vi "Setup-Input-Output-DAQmx.vi"(9 "Sample Rate":dbl=41200.0, 10 "samples per channel":i32=1000, 11 "Accel. 2":bool) -> (0 "error out":errorcluster, 2 "Output task":refnum<k21>, 3 "Input Task":refnum<k21>)   [LabVIEW 2022 SP3]
uses:
  <vilib>/Utility/error.llb/DialogType.ctl
  <vilib>/DAQmx/create/channels.llb/DAQmx Create Channel (AI-Acceleration-Accelerometer).vi
  <vilib>/DAQmx/create/channels.llb/DAQmx Create Channel (AO-Voltage-Basic).vi
  <vilib>/DAQmx/configure/timing.llb/DAQmx Timing (Sample Clock).vi
  <vilib>/DAQmx/configure/trigger.llb/DAQmx Start Trigger (Digital Edge).vi
panel:
  in  "source":tag
  in  "edge":i32(ring)=10280 items=["Rising"=10280, "Falling"=10171]
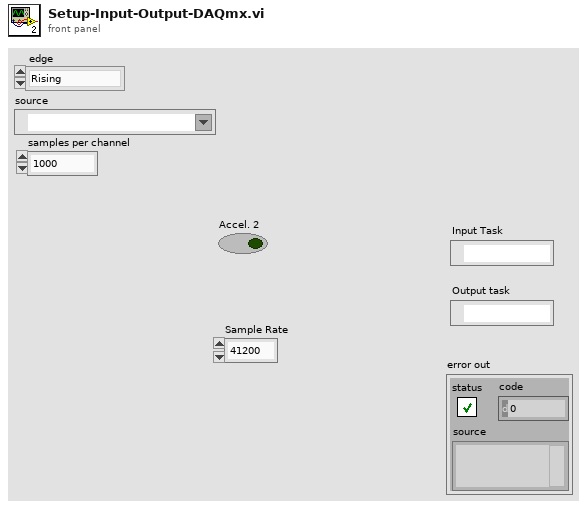
[diagram p1: front panel]
types:
  T1 = typedef "DialogType.ctl" = u16
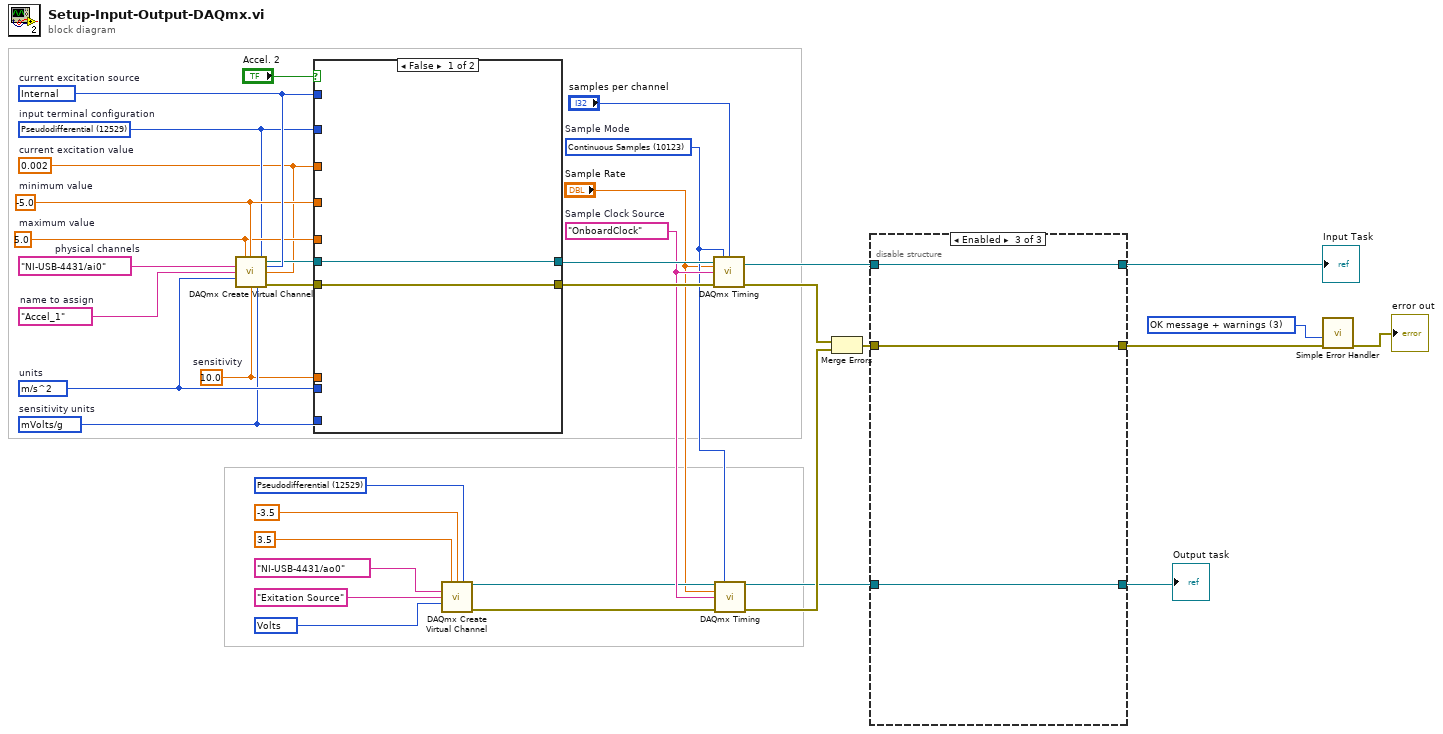
[diagram p0: block diagram]
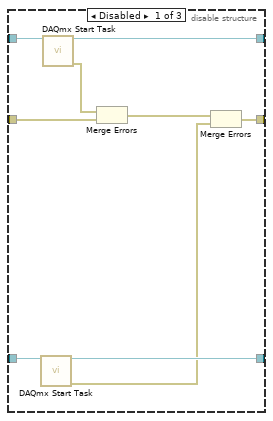
[diagram p2: hidden frame]
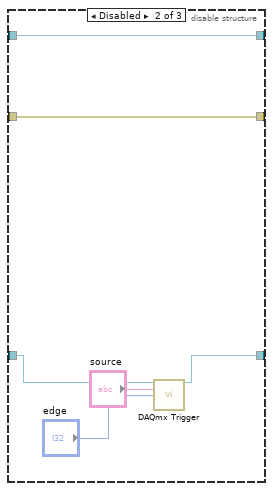
[diagram p3: hidden frame]
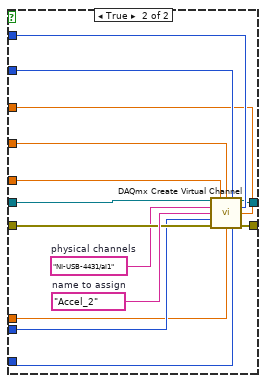
[diagram p4: hidden frame]
diagram:
  w6 = T1 3 items=["no dialog", "OK message", "continue or stop message", "OK message + warnings", "continue/stop + warnings"] ("type of dialog (OK msg:1)")
  w24 = 12529 items=["Default"=-1, "RSE"=10083, "Differential"=10106, "Pseudodifferential"=12529] ("output terminal configuration")
  w22 = 10348 items=["Volts"=10348, "From Custom Scale"=10065] ("units")
  w28 = 12509 items=["mVolts/g"=12509, "Volts/g"=12510]  # sensitivity units
  w20 = 10.0  # sensitivity
  w27 = 0.002  # current excitation value
  w35 = 10200 items=["Internal"=10200, "External"=10167, "None"=10230]  # current excitation source
  w29 = tag "NI-USB-4431/ai0"  # physical channels
  w17 = tag "OnboardClock"  # Sample Clock Source
  w16 = 10123 items=["Finite Samples"=10178, "Continuous Samples"=10123, "Hardware Timed Single Point"=12522]  # Sample Mode
  w31 = 12529 items=["default"=-1, "RSE"=10083, "NRSE"=10078, "Differential"=10106, "Pseudodifferential"=12529]  # input terminal configuration
  w34 = -5.0  # minimum value
  w33 = 5.0  # maximum value
  w37 = "Accel_1"  # name to assign
  w32 = 12470 items=["g"=10186, "m/s^2"=12470, "in/s^2"=12471, "From Custom Scale"=10065]  # units
  n1 = call-poly <vilib>:"DAQmx Create Virtual Channel.vi"("maximum value"=w33, "minimum value"=w34, "input terminal configuration"=w31, "physical channels"=w29, "current excitation source"=w35, "name to assign"=w37, "current excitation value"=w27, "units"=w32, "sensitivity"=w20, "sensitivity units"=w28) -> ("task out"=w30:refnum<k21>, "error out"=w36:errorcluster)  [unwired: 4 in]
  n2 = case shown="False" "Accel. 2" {
    tunnel: w36 -> [w39 w52]
    tunnel: w35 -> [_ w51]
    tunnel: w34 -> [_ w50]
    tunnel: w33 -> [_ w49]
    tunnel: w32 -> [_ w48]
    tunnel: w31 -> [_ w47]
    tunnel: w30 -> [w38 w46]
    tunnel: w28 -> [_ w44]
    tunnel: w27 -> [_ w43]
    tunnel: w20 -> [_ w42]
    tunnel: [w39 w41] -> w19
    tunnel: [w38 w40] -> w18
    frame False {
    }
    frame True {
      w45 = tag "NI-USB-4431/ai1"  # physical channels
      w53 = "Accel_2"  # name to assign
      n3 = call-poly <vilib>:"DAQmx Create Virtual Channel.vi"("task in"=w46, "maximum value"=w49, "minimum value"=w50, "input terminal configuration"=w47, "physical channels"=w45, "current excitation source"=w51, "name to assign"=w53, "current excitation value"=w43, "units"=w48, "error in"=w52, "sensitivity"=w42, "sensitivity units"=w44) -> ("task out"=w40:refnum<k21>, "error out"=w41:errorcluster)  [unwired: 2 in]
    }
  }
  n4 = call-poly <vilib>:"DAQmx Create Virtual Channel.vi"("maximum value"=3.5, "minimum value"=-3.5, "output terminal configuration"=w24, "physical channels"=tag "NI-USB-4431/ao0", "name to assign"="Exitation Source", "units"=w22) -> ("task out"=w14:refnum<k21>, "error out"=w15:errorcluster)  [unwired: 8 in]
  n5 = call-poly <vilib>:"DAQmx Timing.vi"("task/channels in"=w18, "sample mode"=w16, "samples per channel"="samples per channel", "rate"="Sample Rate", "source"=w17, "error in"=w19) -> ("task out"=w10:refnum<k21>, "error out"=w5:errorcluster)  [unwired: 8 in]
  n6 = call-poly <vilib>:"DAQmx Timing.vi"("task/channels in"=w14, "sample mode"=w16, "rate"="Sample Rate", "source"=w17, "error in"=w15) -> ("task out"=w2:refnum<k21>, "error out"=w4:errorcluster)  [unwired: 9 in]
  n7 = Merge Errors(w5, w4) -> (w3:errorcluster)
  n8 = disable-structure shown="Enabled" {
    disable-tunnel: w10 -> [w62 w68 w70]
    disable-tunnel: [w61 w68 w70] -> w9
    disable-tunnel: w2 -> [w60 w66 w71]
    disable-tunnel: [w59 w65 w71] -> w8
    disable-tunnel: [w56 w67 w69] -> w7
    disable-tunnel: w3 -> [w54 w67 w69]
    frame Disabled {
      n9 = call <vilib>:"DAQmx Start Task.vi"("task/channels in"=w60) -> ("task out"=w59:refnum<k21>, "error out"=w55:errorcluster)  [unwired: 13 in]
      n10 = call <vilib>:"DAQmx Start Task.vi"("task/channels in"=w62) -> ("task out"=w61:refnum<k21>, "error out"=w58:errorcluster)  [unwired: 13 in]
      n11 = Merge Errors(w58, w54) -> (w57:errorcluster)
      n12 = Merge Errors(w57, w55) -> (w56:errorcluster)
    }
    frame Disabled {
      n13 = call-poly <vilib>:"DAQmx Trigger.vi"("task/channels in"=w66, "source"="source", "edge"="edge") -> ("task out"=w65:refnum<k21>)  [unwired: 11 in, 1 out]
    }
    frame Enabled {
    }
  }
  "Input Task" <- w9
  "Output task" <- w8
  n14 = call <vilib>:"Simple Error Handler.vi"("type of dialog (OK msg:1)"=w6, "error in (no error)"=w7) -> ("error out"=→"error out":errorcluster)  [unwired: 3 in, 4 out]
